vi "Get NamedUnbundler from Diagram.vi"(11 "Diagram":refnum<vi>) -> (3 "UBN Node":refnum<vi>)   [LabVIEW 2018, in "LVClassByRef.lvlib"]
uses:
  <resource>/Framework/Providers/LVClassByRef/LVClassByRef.lvlib
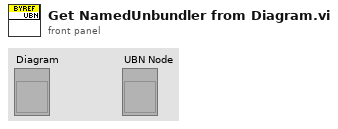
[diagram p1: front panel]
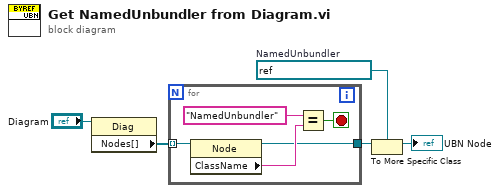
[diagram p0: block diagram]
diagram:
  w3 = refnum<vi> refnum  # NamedUnbundler
  n1 = property class="Diag"(reference="Diagram") -> ("Nodes[]"=w5:refnum<vi>[])  [unwired: 1 in, 2 out]
  n2 = for {
    tunnel: w5 -> [w10] mode=indexing
    tunnel: [w6] -> w4
    stop <- w7 stop-if-true
    n3 = property class="Node"(reference=w10) -> (reference out=w6:refnum<vi>, "ClassName"=w8:string)  [unwired: 1 in, 1 out]
    n4 = Equal?(x="NamedUnbundler", y=w8) -> (x = y?=w7:bool)
  }
  n5 = To More Specific Class(target class=w3, reference=w4) -> (specific class reference=→"UBN Node":refnum<vi>)  [unwired: 1 in, 1 out]
